vi "MeasureTransconductance.vi"(0 ".NET Refnum in":refnum<k24>, 1 "UiDefinition":T1, 2 "Junction Name":string, 5 ".NET Refnum":refnum<k24>, 7 "appended path":path, 9 "Path":path, 12 "new file path (Not A Path if cancelled)":path, 13 "Function":string) -> (4 "Cluster":cluster{dbl[], dbl[]}, 15 "error out":errorcluster)   [LabVIEW 2020]
uses:
  UIReferences.ctl
  D:/LabviewDXFViewer/LabviewDXFViewer/bin/Release/LabviewDXFViewer.exe
  LabviewDXFViewer/bin/Release/LabviewDXFViewer.exe
  <vilib>/Utility/file.llb/Write Delimited Spreadsheet (DBL).vi
  <vilib>/Utility/file.llb/Write Delimited Spreadsheet (string).vi
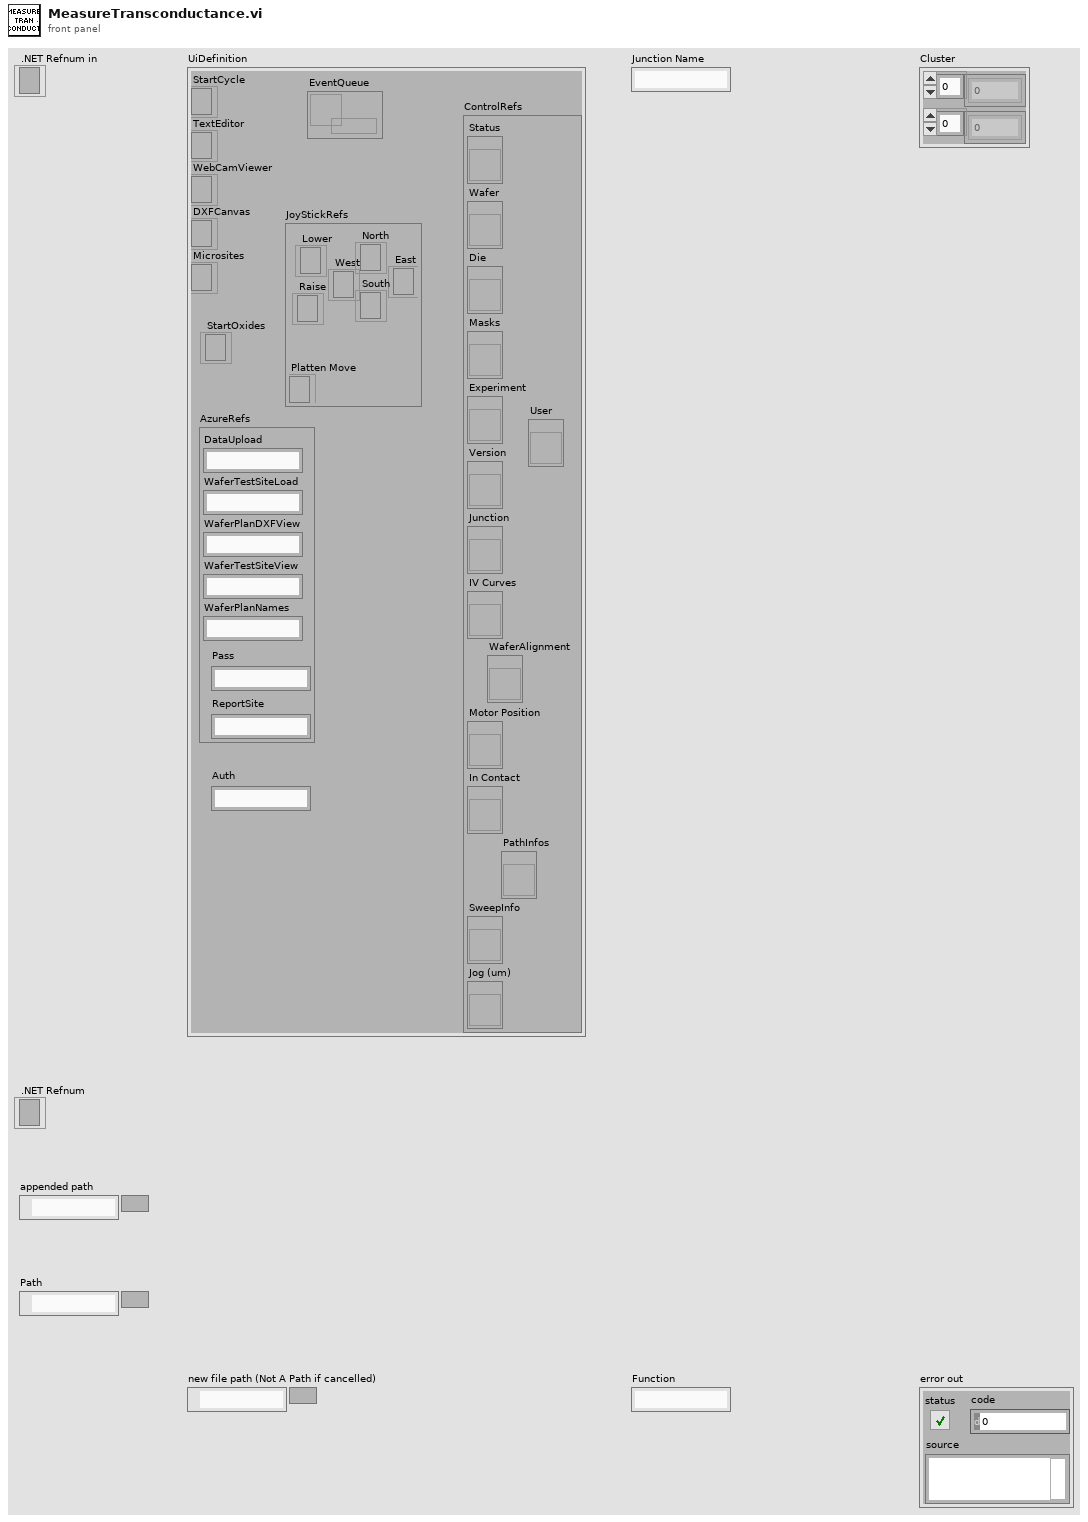
[diagram p1: front panel]
types:
  T1 = typedef "UIReferences.ctl" = cluster{"StartCycle":refnum<k24>, "TextEditor":refnum<k24>, "WebCamViewer":refnum<k24>, "DXFCanvas":refnum<k24>, "Microsites":refnum<k24>, "JoyStickRefs":cluster{"North":refnum<k24>, "Lower":refnum<k24>, "Raise":refnum<k24>, "Platten Move":refnum<k24>, "West":refnum<k24>, "East":refnum<k24>, "South":refnum<k24>}, "AzureRefs":cluster{"DataUpload":string, "WaferTestSiteLoad":string, "WaferPlanDXFView":string, "WaferTestSiteView":string, "WaferPlanNames":string, "Pass":string, "ReportSite":string}, "ControlRefs":cluster{"Status":refnum<vi>, "Wafer":refnum<vi>, "Die":refnum<vi>, "Masks":refnum<vi>, "Experiment":refnum<vi>, "Version":refnum<vi>, "Junction":refnum<vi>, "IV Curves":refnum<vi>, "Motor Position":refnum<vi>, "In Contact":refnum<vi>, "SweepInfo":refnum<vi>, "Jog (um)":refnum<vi>, "PathInfos":refnum<vi>, "User":refnum<vi>, "WaferAlignment":refnum<vi>}, "EventQueue":refnum<queue>, "StartOxides":refnum<k24>, "Auth":string}
  T2 = typedef "CapacitanceInfos.ctl" = cluster{"Conductance":dbl, "CapacitanceIV":dbl, "Intercept":dbl, "CapacitanceSW":dbl, "Sum":dbl, "CapacitanceInfos":T3[], "CapacitancePhase":dbl, "dC/dV":dbl, "Function":string, "OtherInfo":dbl[][]}
  T3 = typedef "CapacitanceRecord.ctl" = cluster{"Freq":dbl, "Vpp":dbl, "PhaseS":dbl, "Irms":dbl, "PhaseC":dbl, "Theta":dbl, "VDrive":dbl, "Capacitance":dbl, "Other":dbl}
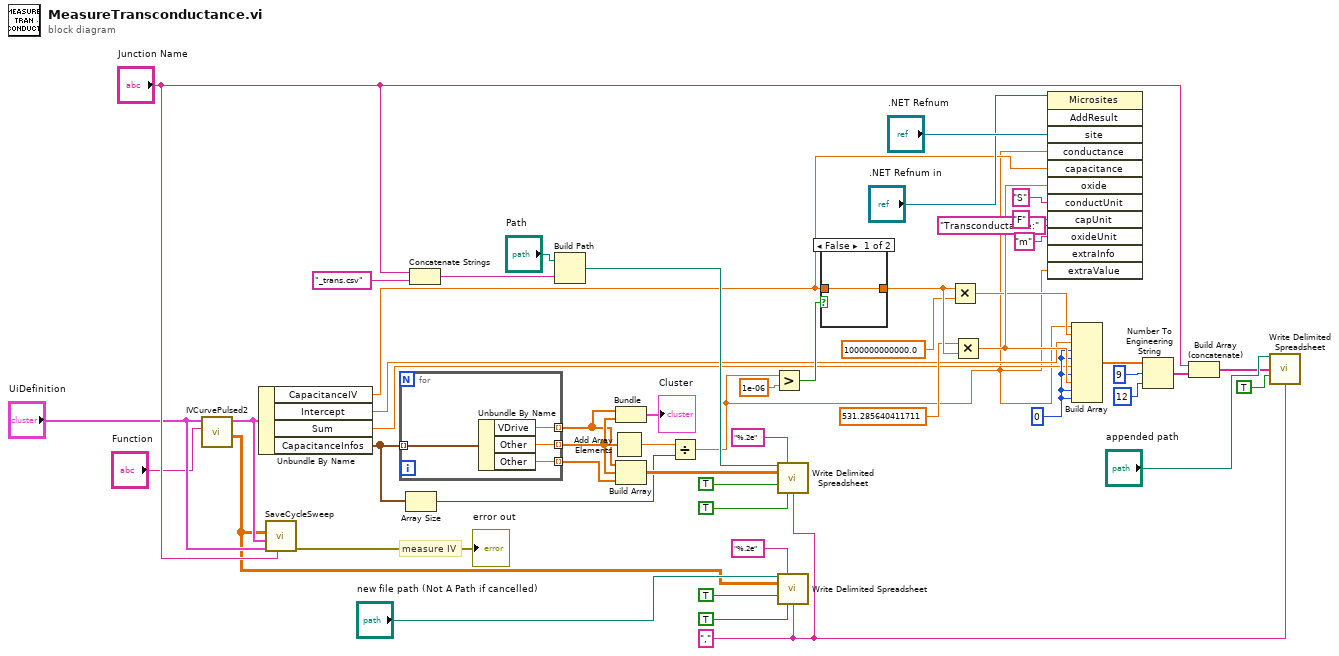
[diagram p0: block diagram]
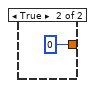
[diagram p2: hidden frame]
diagram:
  w3 = "," ("delimiter (\\t)")
  w25 = 0
  # "measure IV"
  n1 = call "IVCurvePulsed2.vi"("Program"="Function", "UiDefinition"="UiDefinition") -> ("appended array"=w11:dbl[][], "InfoCluster"=w24:T2)  [unwired: 8 in]
  n2 = Unbundle By Name(w24) -> ("CapacitanceIV"=w26:dbl, "Intercept"=w14:dbl, "Sum"=w15:dbl, "CapacitanceInfos"=w35:T3[])
  n3 = call "SaveCycleSweep.vi"("JunctionName"="Junction Name", "UiDefinition 2"="UiDefinition", "InfoCluster"=w24, "appended array"=w11) -> ("error out"=→"error out":errorcluster)  [unwired: 7 in]
  n4 = for {
    tunnel: w35 -> [w55] mode=indexing
    tunnel: [w54] -> w48 mode=indexing
    tunnel: [w53] -> w49 mode=indexing
    tunnel: [w52] -> w50 mode=indexing
    n5 = Unbundle By Name(w55) -> ("VDrive"=w54:dbl, "Other"=w53:dbl, "Other"=w52:dbl)
  }
  n6 = Array Size(array=w35) -> (size(s)=w34:i32)
  n7 = Concatenate Strings("Junction Name", "_trans.csv" ("string")) -> (w41:string)
  n8 = Build Path(base path="Path", name or relative path=w41) -> (appended path=w47:path)
  n9 = Add Array Elements(numeric array=w49) -> (sum=w33:dbl)
  n10 = Bundle(w48, w49) -> (→"Cluster":cluster{dbl[], dbl[]})  [unwired: 1 in]
  n11 = Build Array(w48, w49, w50) -> (w51:dbl[][])
  n12 = Divide(x=w33, y=w34) -> (x/y=w2:dbl)
  n13 = Greater?(x=w2, y=1e-06) -> (0:w18:bool)
  n14 = call-poly <vilib>:"Write Delimited Spreadsheet.vi"("file path (dialog if empty)"=w47, "format (%.3f)"="%.2e", "2D data"=w51, "append to file? (new file:F)"=TRUE, "transpose? (no:F)"=TRUE, "delimiter (\\t)"=w3) -> ()  [unwired: 8 in, 2 out]
  n15 = call-poly <vilib>:"Write Delimited Spreadsheet.vi"("file path (dialog if empty)"="new file path (Not A Path if cancelled)", "format (%.3f)"="%.2e", "2D data"=w11, "append to file? (new file:F)"=TRUE, "transpose? (no:F)"=TRUE, "delimiter (\\t)"=w3) -> ()  [unwired: 8 in, 2 out]
  n16 = case shown="False" w18 {
    tunnel: [w56 0] -> w37
    tunnel: w26 -> [w56 _]
    frame False {
    }
    frame True {
    }
  }
  n17 = Multiply(x=w37, y=1000000000000.0) -> (x*y=w16:dbl)
  n18 = Multiply(x=531.285640411711, y=w37) -> (x*y=w38:dbl)
  n19 = invoke class="Microsites" method="AddResult"(reference=".NET Refnum in", "site"=".NET Refnum", "conductance"=w2, "capacitance"=w26, "oxide"=w38, "conductUnit"="S", "capUnit"="F", "oxideUnit"="m" ("interceptUnit"), "extraInfo"="Transconductance:", "extraValue"=w2) -> ()  [unwired: 2 in, 12 out]
  n20 = Build Array(w2, w16, w14, w25, w25, w15, w25, w38, w25, w25) -> (w13:dbl[])
  n21 = Number To Engineering String(2:i16 12 ("precision (6)"), 3:i16 9 ("width (-)"), 4:w13) -> (0:w5:string[])  [unwired: 1 in]
  n22 = Build Array (concatenate)("Junction Name", w5) -> (w7:string[])
  n23 = call-poly <vilib>:"Write Delimited Spreadsheet.vi"("file path (dialog if empty)"="appended path", "1D data"=w7, "append to file? (new file:F)"=TRUE, "delimiter (\\t)"=w3) -> ()  [unwired: 10 in, 2 out]
